vi "Configuration_Ref_API.vi"(0 "DVR In":refnum<data-value>, 11 "Error In":errorcluster) -> (4 "DVR Out":refnum<data-value>, 6 "VI Ref":refnum<vi>, 8 "Configuration Ref":refnum<vi>, 15 "Error Out":errorcluster)   [LabVIEW 2020, in "Test.lvclass"]
uses:
  Test.lvclass
  Children/INL DNL Test/INL DNL Test.lvclass
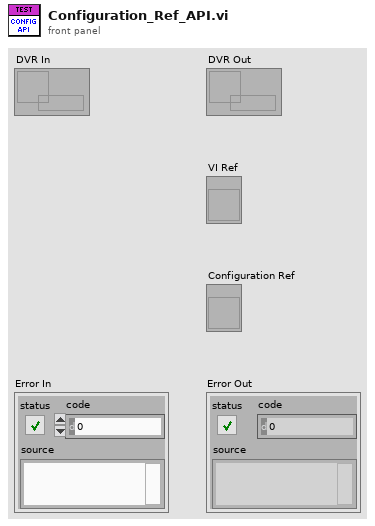
[diagram p1: front panel]
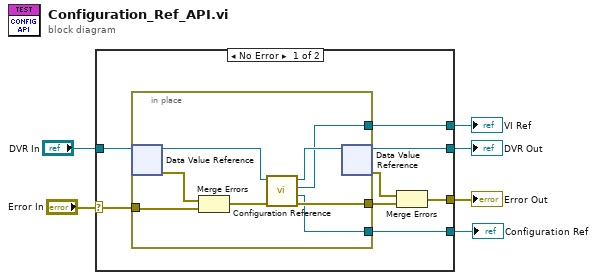
[diagram p0: block diagram]
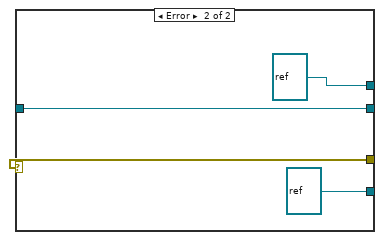
[diagram p2: hidden frame]
diagram:
  n1 = case shown="No Error" "Error In" {
    selector: "Error In" -> [w13 w26]
    tunnel: "DVR In" -> [w14 w25]
    tunnel: [w12 refnum<vi> refnum ("VI Ref")] -> w4
    tunnel: [w11 w25] -> w3
    tunnel: [w8 w26] -> w2
    tunnel: [w7 refnum<vi> refnum ("Configuration Ref")] -> w1
    frame No Error {
      n2 = in-place {
        in-place-border: w13 -> [w22]
        in-place-border: [w17] -> w12
        in-place-border: [w16] -> w9
        in-place-border: [w15] -> w7
        n3 = in-place-dvr #1(w14) -> (w19:refnum<class "Test.lvclass">, w21:errorcluster)
        n4 = Merge Errors(w21, w22) -> (w20:errorcluster)
        n5 = call-dynamic "Configuration Reference.vi"("Error in"=w20, "Test in"=w19) -> ("Error out"=w16:errorcluster, "Configuration Ref"=w15:refnum<vi>, "VI Ref"=w17:refnum<vi>, "Test out"=w18:refnum<class "Test.lvclass">)  [unwired: 6 in]
        n6 = in-place-dvr #1(w18) -> (w11:refnum<data-value>, w10:errorcluster)
      }
      n7 = Merge Errors(w10, w9) -> (w8:errorcluster)
    }
    frame Error {
    }
  }
  "VI Ref" <- w4
  "DVR Out" <- w3
  "Error Out" <- w2
  "Configuration Ref" <- w1
